vi "SS_PulseInfo.vi"(6 "Main Cluster IN":T1, 8 "Error In":errorcluster, 11 "Info In":string="\nWaiting for TimerScope Trigger\n- IN: SS TimerScope Trigger\n- OUT: SET SS ThermoRec Received Trigger\nPulse Number is 231123\nPulse Type is 4\n\nDuration (s) is  2.000000\nDelay (s)  is  1.000000\nScan Period (ms) is  15\nNumber of Samples is  134\n\nDelay Started\nDelay Complete\nExternal Measurement of Delay (s): 1.000000\nACQUIRING DATA") -> (0 "Error Out":errorcluster, 3 "Info Out":string="\nWaiting for TimerScope Trigger\n- IN: SS TimerScope Trigger\n- OUT: SET SS ThermoRec Received Trigger\nPulse Number is 231123\nPulse Type is 4\n\nDuration (s) is  2.000000\nDelay (s)  is  1.000000\nScan Period (ms) is  15\nNumber of Samples is  134\n\nDelay Started\nDelay Complete\nExternal Measurement of Delay (s): 1.000000\nACQUIRING DATA", 4 "Main Cluster OUT":T1)   [LabVIEW 2016]
uses:
  Control/Control_Main.ctl
  Control/Control_ModuleArray.ctl
panel:
  in  "Tab Control":enum32{"IN", "OUT", "SubVI Info"}(tab)
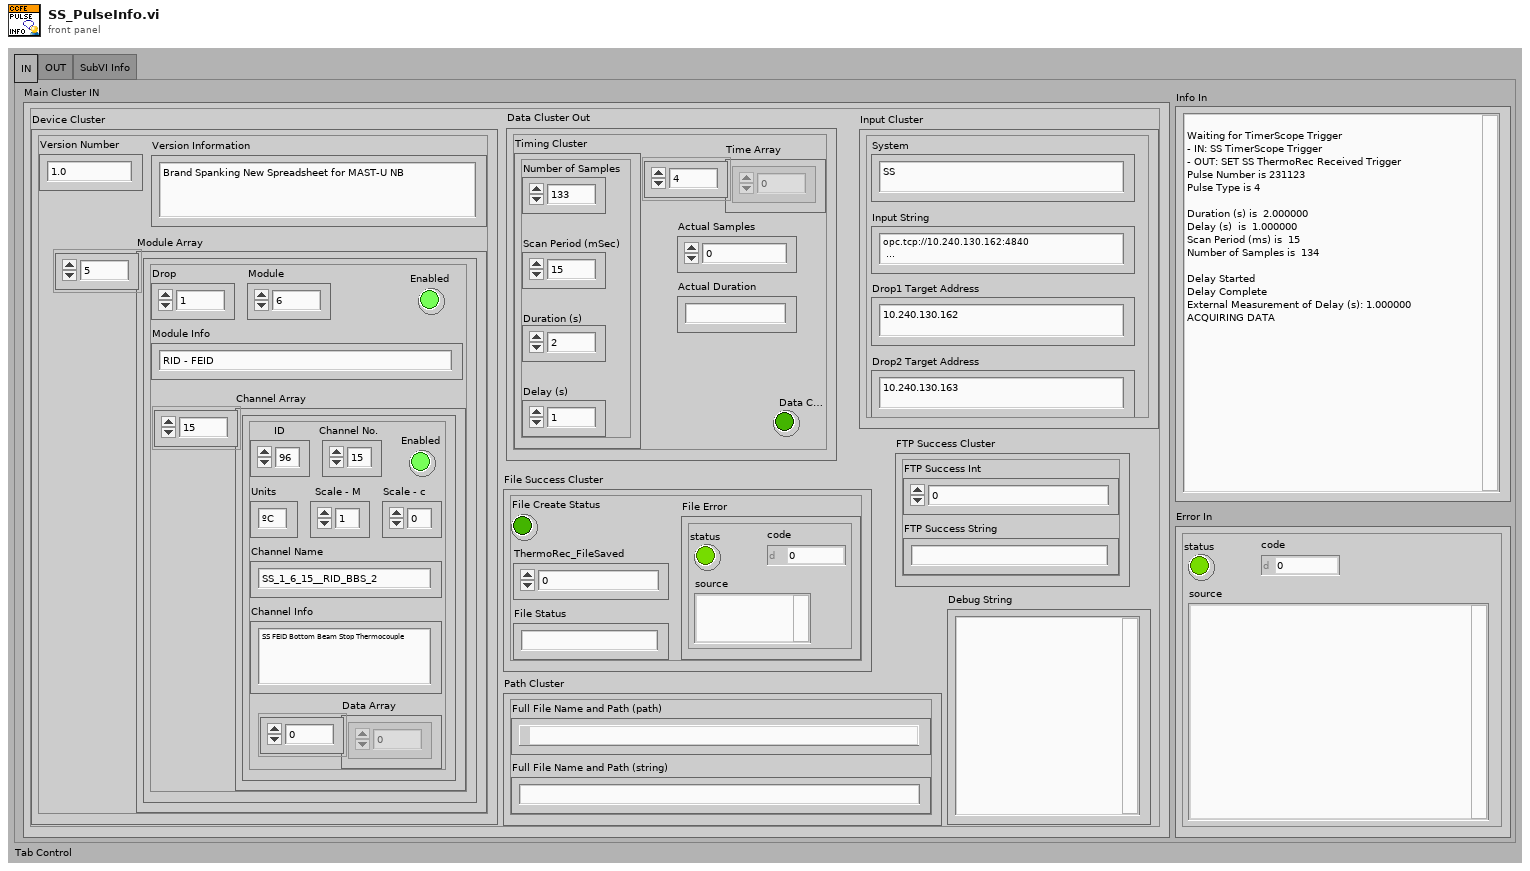
[diagram p1: front panel]
types:
  T1 = typedef "Control_Main.ctl" = cluster{"Device Cluster":cluster{"Module Array":T2, "Version Number":string, "Version Information":string}, "Input Cluster":cluster{"Input String":string, "Drop1 Target Address":string, "Drop2 Target Address":string, "System":string}, "Data Cluster Out":cluster{"Timing Cluster":cluster{"Number of Samples":i32, "Scan Period (mSec)":u32, "Duration (s)":dbl, "Delay (s)":dbl}, "Time Array":dbl[], "Actual Samples":i32, "Actual Duration":string, "Data Collection Error":bool}, "Path Cluster":cluster{"Full File Name and Path (path)":path, "Full File Name and Path (string)":string}, "File Success Cluster":cluster{"ThermoRec_FileSaved":i32, "File Create Status":bool, "File Error":errorcluster, "File Status":string}, "FTP Success Cluster":cluster{"FTP Success Int":i32, "FTP Success String":string}, "Debug String":string}
  T2 = typedef "Control_ModuleArray.ctl" = cluster{"Drop":i32, "Module":i32, "Module Info":string, "Enabled":bool, "Channel Array":cluster{"ID":i32, "Channel No.":i32, "Enabled":bool, "Channel Name":string, "Channel Info":string, "Units":string, "Scale - M":dbl, "Scale - c":dbl, "Data Array":dbl[]}[]}[]
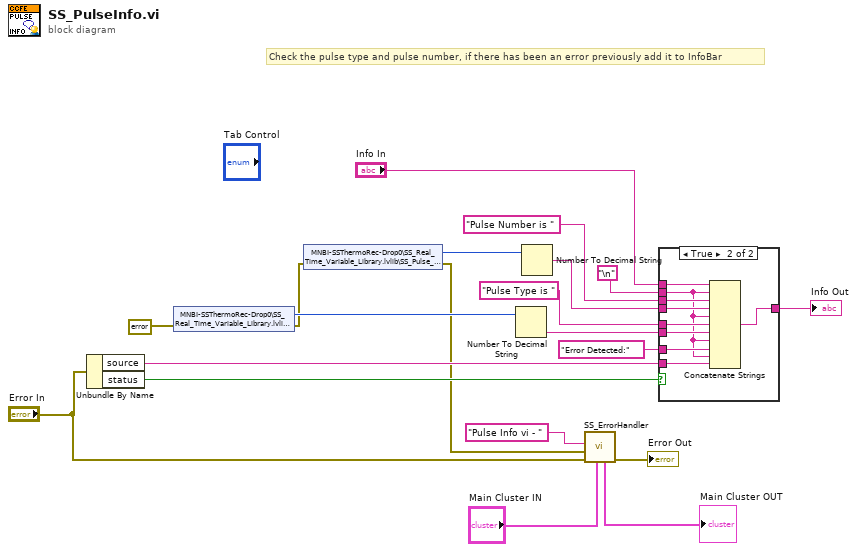
[diagram p0: block diagram]
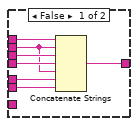
[diagram p2: hidden frame]
diagram:
  # "Check the pulse type and pulse number, if there has been an error previously add it to InfoBar"
  n1 = Unbundle By Name("Error In") -> ("source"=w20:string, "status"=w18:bool)
  n2 = shared-variable "MNBI-SSThermoRec-Drop0\\SS_Real_Time_Variable_Library.lvlib\\SS_Pulse_Type"(error in=errorcluster {"status"=FALSE, "code"=0, "source"=""} ("error constant")) -> (w11:i32, error out=w10:errorcluster)
  n3 = shared-variable "MNBI-SSThermoRec-Drop0\\SS_Real_Time_Variable_Library.lvlib\\SS_Pulse_Number"(error in=w10) -> (w12:i32, error out=w1:errorcluster)
  n4 = Number To Decimal String(number=w11) -> (decimal integer string=w16:string)  [unwired: 1 in]
  n5 = Number To Decimal String(number=w12) -> (decimal integer string=w15:string)  [unwired: 1 in]
  n6 = call "SS_ErrorHandler.vi"("Main Cluster IN"="Main Cluster IN", "Error In"="Error In", "SubVI Error"=w1, "SubVI Name"="Pulse Info vi - ") -> ("Error Out"=→"Error Out":errorcluster, "Main Cluster OUT"=→"Main Cluster OUT":T1)  [unwired: 5 in, 1 out]
  n7 = case shown="True" w18 {
    tunnel: "Pulse Type is " -> [w27 w36]
    tunnel: "Pulse Number is " -> [w26 w35]
    tunnel: w15 -> [w25 w34]
    tunnel: w16 -> [w24 w33]
    tunnel: [w23 w32] -> w7
    tunnel: "Info In" -> [w22 w31]
    tunnel: "\n" -> [w21 w29]
    tunnel: "Error Detected:" -> [_ w30]
    tunnel: w20 -> [_ w28]
    frame False {
      n8 = Concatenate Strings(w22, w21, w26, w25, w21, w27, w24) -> (w23:string)
    }
    frame True {
      n9 = Concatenate Strings(w31, w29, w35, w34, w29, w36, w33, w29, w30, w29, w28) -> (w32:string)
    }
  }
  "Info Out" <- w7
